vi "AB_Set_TargetFile_Name.vi"(8 "error in (no error)":errorcluster, 10 "Target filename":string, 11 "TargetFile in":refnum<class "AB_Targetfile.lvclass">) -> (0 "error out":errorcluster, 3 "TargetFile out":refnum<class "AB_Targetfile.lvclass">)   [LabVIEW 2020]
uses:
  <vilib>/AppBuilder/AB_Classes/TargetFile/AB_Targetfile.lvclass
  e:/builds/penguin/labview/branches/2020/dev/dist/vi.lib/AppBuilder/AB_Classes/Build/AB_Build.lvclass
  <vilib>/AppBuilder/AB_Classes/Build/AB_Build.lvclass
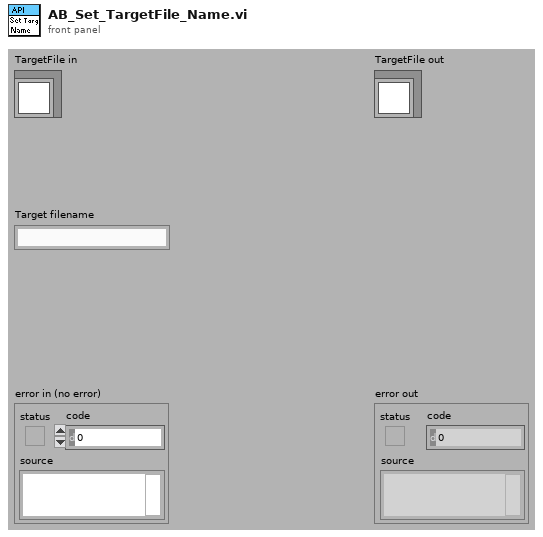
[diagram p1: front panel]
types:
  T1 = typedef "AB_Targetfile.ctl" = cluster{"targetfileName":string, "targetfileGUID":string, "enableDebugging":bool, "versionInfo":cluster{"productName":string, "legalCopyright":string, "companyName":string, "internalName":string, "fileDescription":string}, "eng_consolidatedTypeInfo":string, "fastFileFormat":bool, "eng_LEIFBuildData":u32, "versionIndependent":bool}
  T2 = typedef "AB_Build.ctl" = cluster{"buildSpecName":string, "buildSpecDescription":string, "destinations":refnum<class "AB_Destination.lvclass">[], "exclusionOption":T3, "defaultLanguage":string, "supportedLanguages":string[], "excludedDirectories":path[], "buildContext":refnum<vi>, "buildObject":T4, "preview":bool, "programatic":bool, "progressBarEvents":T5, "userLog_Path":path, "preActionID":string, "preAction_Path":path, "postActionID":string, "postAction_Path":path, "eng_checkForBrokenVIs?":bool, "eng_verboseLinkerErrors?":bool, "localDest_Path":path, "targetDest_Path":path, "removeVIObject":u16, "cache":refnum<class "PreviewCache.lvclass">, "use cache":bool, "previewCache_ID":string, "buildCache_ID":string, "eng_TempLocalDest_Path":path, "eng_collectDependencies?":bool, "versionInfo":cluster{"buildVersion":cluster{"major":u16, "minor":u16, "patch":u16, "build":u16}, "autoIncrement":bool}, "eng_enableVIChecksums":bool}
  T3 = typedef "AB_Exclusion_Option.ctl" = cluster{"typedefs":bool, "polymorphicVIs":bool, "unusedLibraryItems":bool, "modifyLibraryFile":bool, "edit-timeDependencies":bool, "inlineVIs":bool, "dependent PPLs":bool, "dependent DLLs":bool}
  T4 = typedef "ItemRef.ctl" = u64
  T5 = typedef "provcom_ProgressBar_Events.ctl" = cluster{"newJob":refnum<user-event>, "newItem":refnum<user-event>, "errorMsg":T6, "cancel":refnum<user-event>}
  T6 = typedef "mxLvBuildError.ctl" = refnum<user-event>
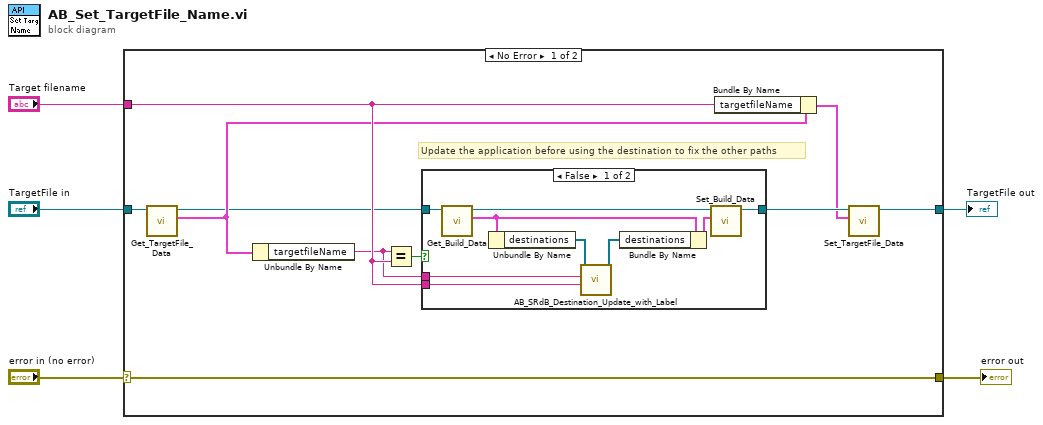
[diagram p0: block diagram]
diagram:
  n1 = case shown="No Error" "error in (no error)" {
    selector: "error in (no error)" -> [w15 w27]
    tunnel: [w15 w27] -> w4
    tunnel: [w10 w26] -> w3
    tunnel: "TargetFile in" -> [w8 w26]
    tunnel: "Target filename" -> [w13 _]
    frame No Error {
      # "Update the application before using the destination to fix the other paths"
      n2 = call <vilib>:"Get_TargetFile_Data.vi"("AB_Targetfile in"=w8) -> ("data"=w9:T1, "AB_Targetfile out"=w7:refnum<class "AB_Targetfile.lvclass">)  [unwired: 8 in, 1 out]
      n3 = Unbundle By Name(w9) -> ("targetfileName"=w12:string)
      n4 = Equal?(x=w12, y=w13) -> (x = y?=w14:bool)
      n5 = case shown="False" w14 {
        tunnel: w13 -> [w23 _]
        tunnel: w12 -> [w24 _]
        tunnel: w7 -> [w22 w25]
        tunnel: [w16 w25] -> w11
        frame False {
          n6 = call <vilib>:"Get_Build_Data.vi"("Class in"=w22) -> ("data"=w20:T2, "Class out"=w18:refnum<class "AB_Targetfile.lvclass">)  [unwired: 1 in, 8 out]
          n7 = Unbundle By Name(w20) -> ("destinations"=w21:refnum<class "AB_Destination.lvclass">[])
          n8 = call <resource>:"AB_SRdB_Destination_Update_with_Label.vi"("new label"=w23, "old label"=w24, "ALL data in"=w21) -> ("ALL data out"=w19:refnum<class "AB_Destination.lvclass">[])  [unwired: 1 in, 7 out]
          n9 = Bundle By Name(cluster=w20, "destinations"=w19) -> (w17:T2)
          n10 = call <vilib>:"Set_Build_Data.vi"("data"=w17, "Class in"=w18) -> ("Class out"=w16:refnum<class "AB_Targetfile.lvclass">)  [unwired: 1 in, 8 out]
        }
        frame True {
        }
      }
      n11 = Bundle By Name(cluster=w9, "targetfileName"=w13) -> (w6:T1)
      n12 = call <vilib>:"Set_TargetFile_Data.vi"("data"=w6, "AB_Targetfile in"=w11) -> ("AB_Targetfile out"=w10:refnum<class "AB_Targetfile.lvclass">)  [unwired: 8 in, 1 out]
    }
    frame Error {
    }
  }
  "error out" <- w4
  "TargetFile out" <- w3
